vi "UPS_Monitor.vi"() -> ()   [LabVIEW 2021]
doc: "This is the Main VI that performs the UPS and capture data from DAQ and simulate the UPS"
uses:
  Controls/Queue_Operation_Select.ctl
  Controls/Acquired_Data.ctl
  Controls/State_and_Data.ctl
  Controls/Acquired_Datactl_Display.ctl
  Controls/File_Operation_Select.ctl
  Controls/UPS_Data.ctl
  Controls/Notifier_Operation_Select.ctl
  Controls/Error_Data.ctl
panel:
  out "Error_Out":errorcluster
  in  "Error_In":errorcluster
  in  "Tab Control":enum32{"PARAMETER", "DETAILS"}(tab)
  out "ACQUIRED_DATA":T1 {"Power_Consumption" scale=0.0..10.0; "Battery_Power" scale=0.0..100.0}
  out "Low_Power_Indicator":bool caption="Low Power Indicator"
  out "Waveform Graph":dbl[][](graph)
  in  "Record":bool
  in  "Stop":bool
  in  "Pause":bool
  in  "Start":bool
  # "UPS Monitor"
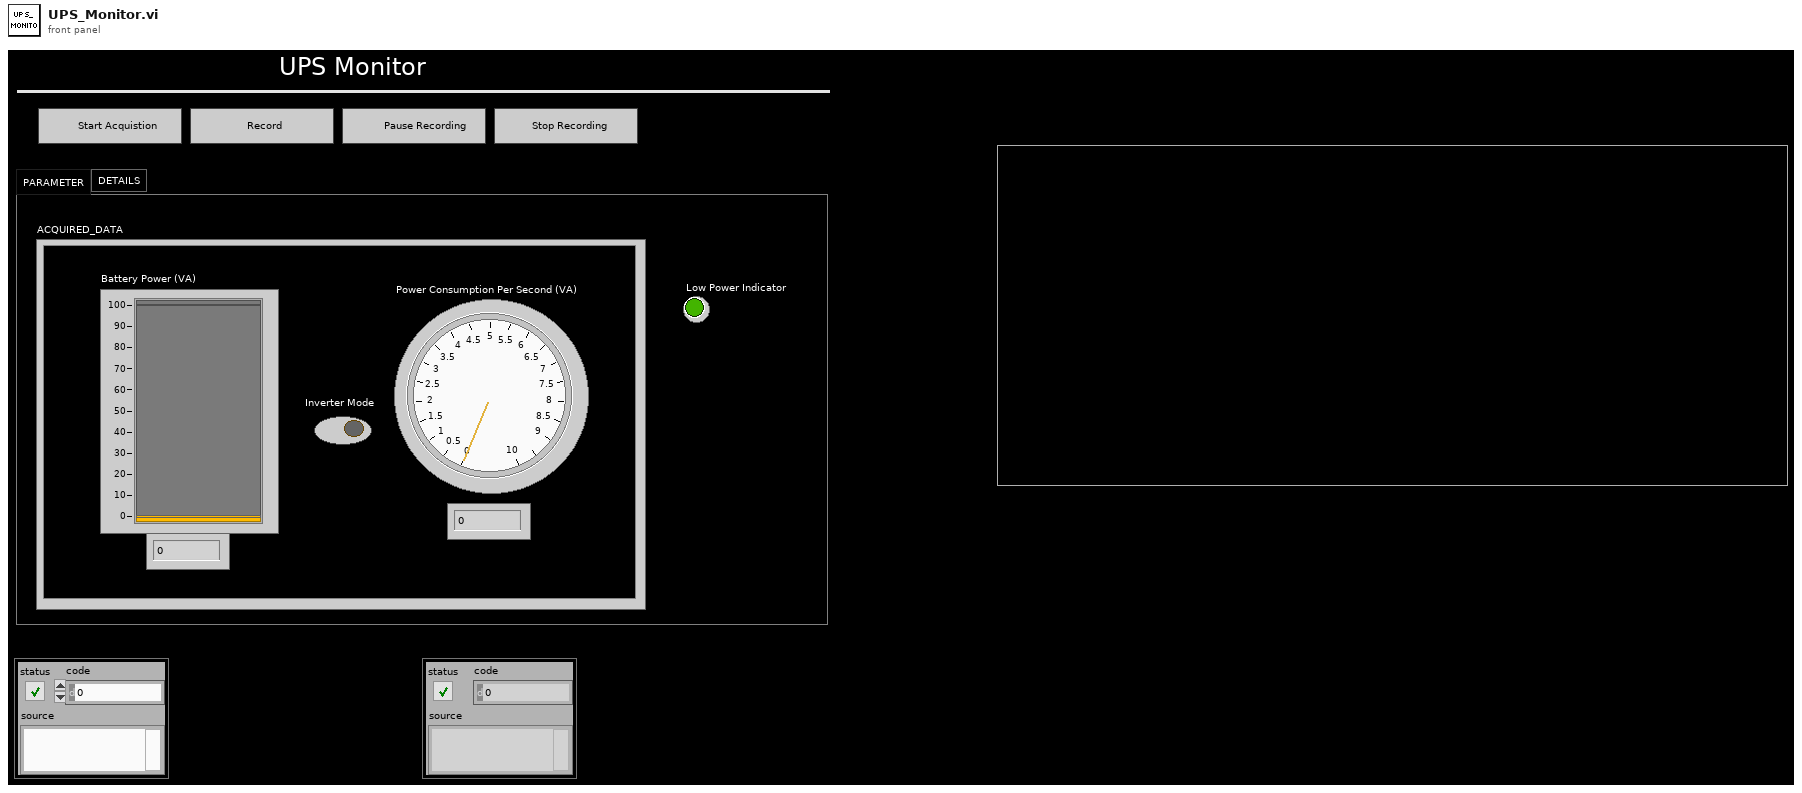
[diagram p1: front panel]
types:
  T1 = typedef "Acquired_Datactl_Display.ctl" = cluster{"Battery_Power":dbl, "Power_Consumption":dbl, "Inverter_Mode":bool}
  T2 = typedef "File_Operation_Select.ctl" = enum16{"Open", "Write", "Read", "Close"}
  T3 = typedef "Queue_Operation_Select.ctl" = enum16{"Obtain_Queue", "Enqueue", "Enqueue_First", "Enqueue_N", "Lossy_Enqueue", "Preview", "Queue_Status", "Dequeue", "Flush", "Release_Queue"}
  T4 = typedef "Notifier_Operation_Select.ctl" = enum16{"Obtain_Notifier", "Send_Notification", "Get_Notifier_Status", "Release_Notifier"}
  T5 = typedef "State_and_Data.ctl" = cluster{"State":string, "Data":variant}
  T6 = typedef "UPS_Data.ctl" = cluster{"ACQUIRED_DATA":T7, "Start":bool, "Pause":bool, "Record":bool, "Low_Power":bool, "Power_and_Power_Consumed":dbl[][], "State_and_Data_In":T5, "File_Path":path, "Application_Directory":path, "Record_Select":enum8{"Enabled", "Disabled", "Disabled and Grayed Out"}, "Stop_Select":enum8{"Enabled", "Disabled", "Disabled and Grayed Out"}}
  T7 = typedef "Acquired_Data.ctl" = cluster{"Battery_Power":dbl, "Power_Consumption":dbl, "Inverter_Mode":bool}
  T8 = enum8{"Enabled", "Disabled", "Disabled and Grayed Out"}
  T9 = typedef "Error_Data.ctl" = cluster{"Module_Name":string, "Error":errorcluster}
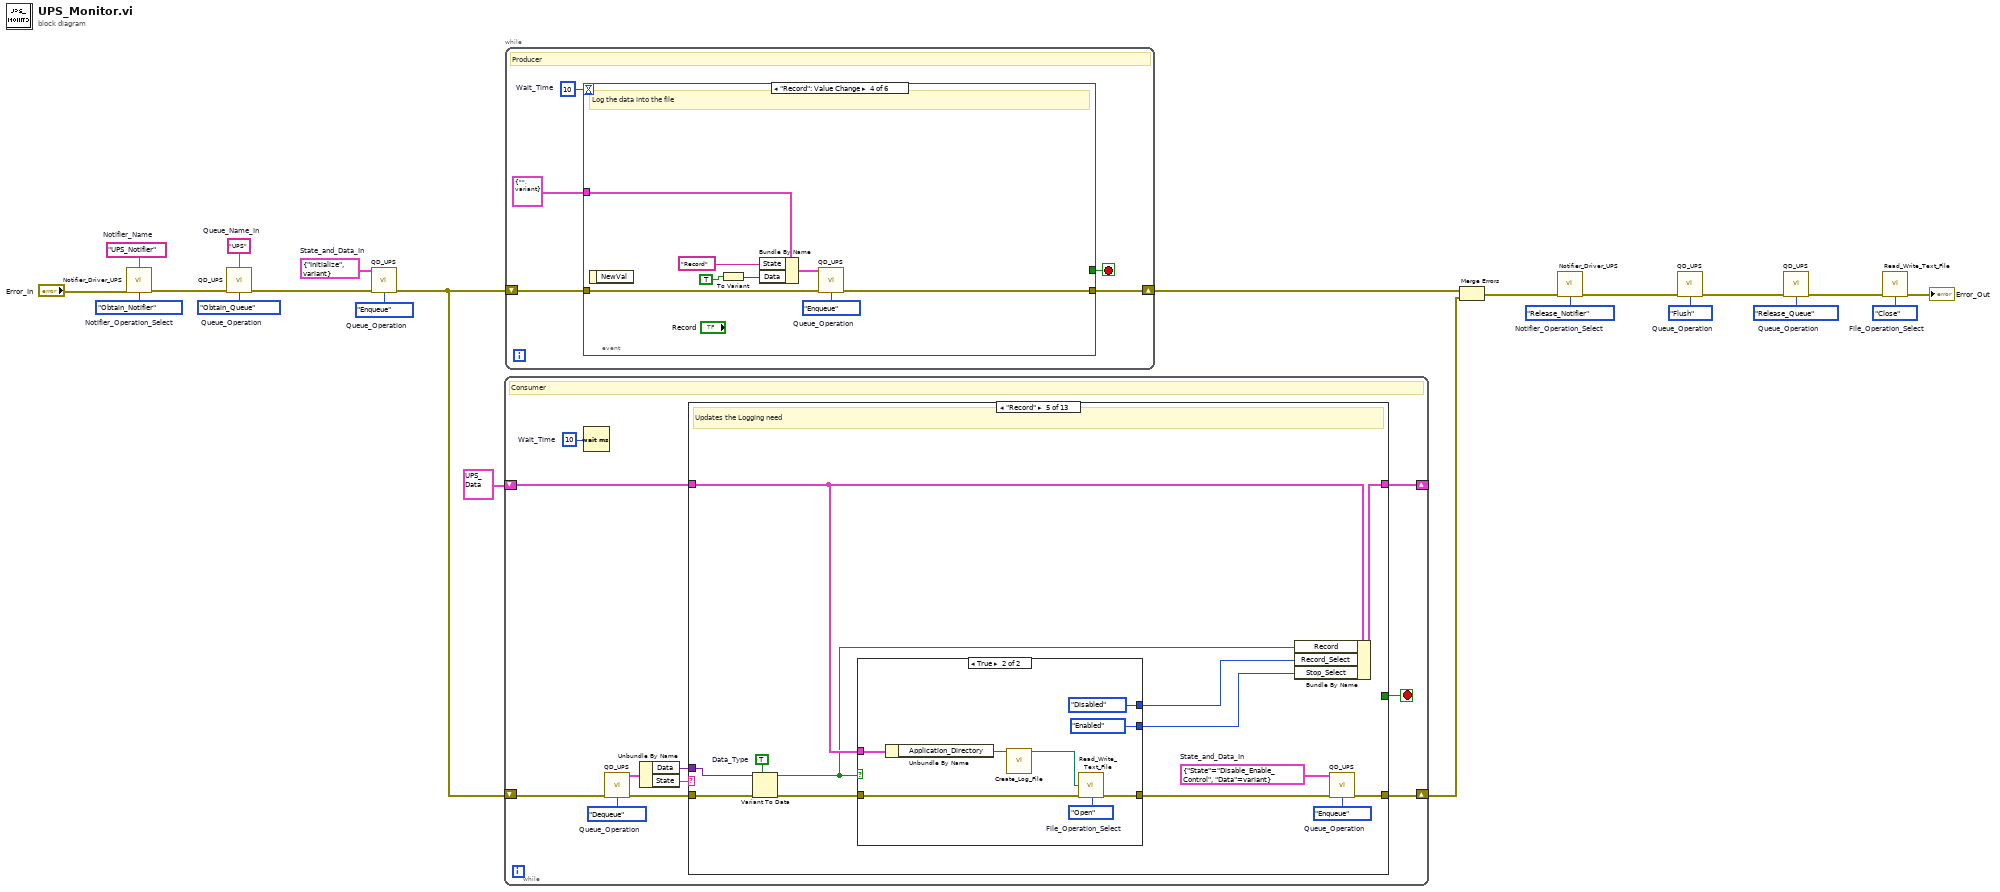
[diagram p0: block diagram]
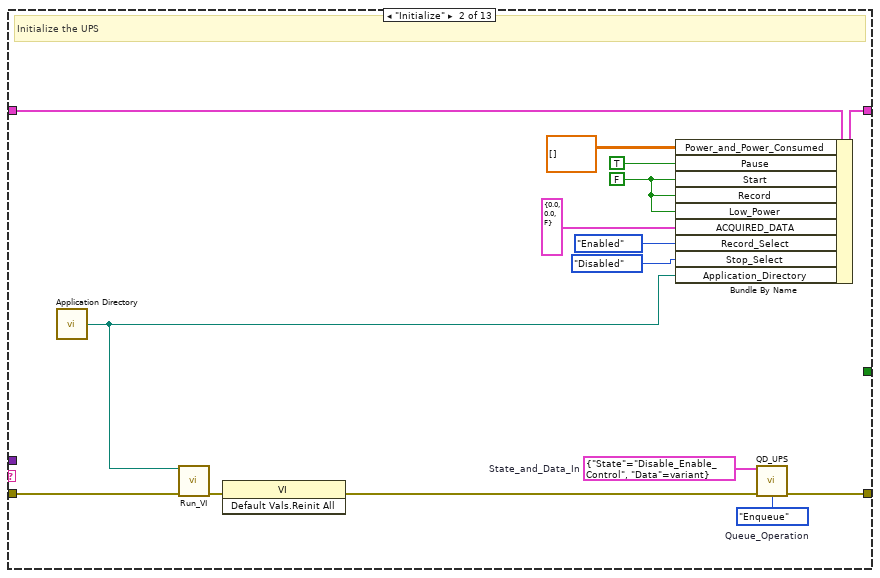
[diagram p3: hidden frame]
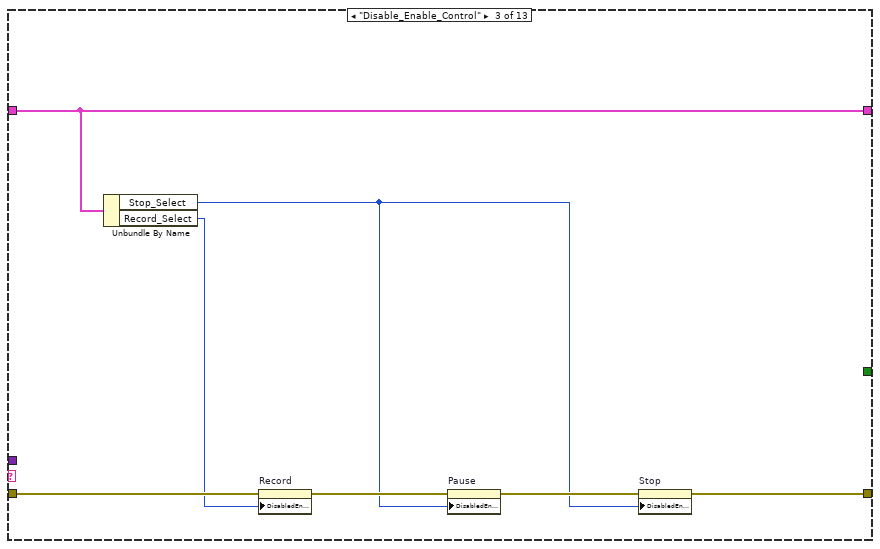
[diagram p4: hidden frame]
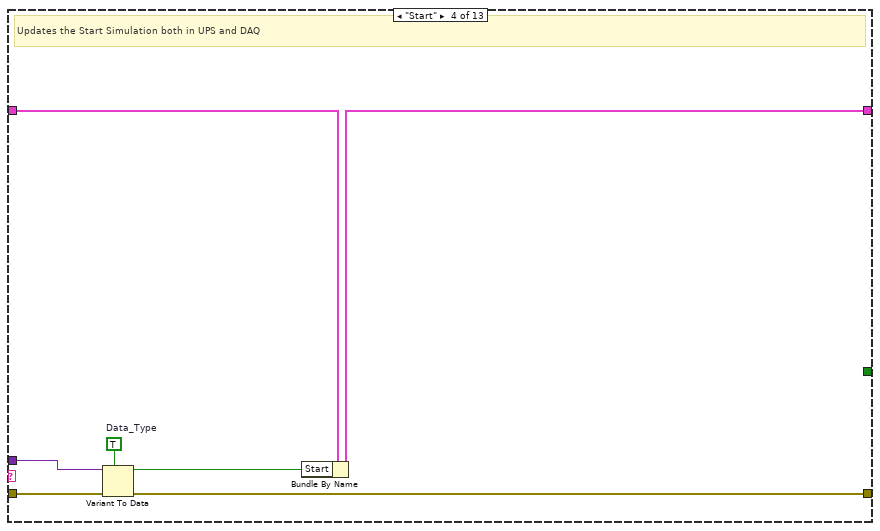
[diagram p5: hidden frame]
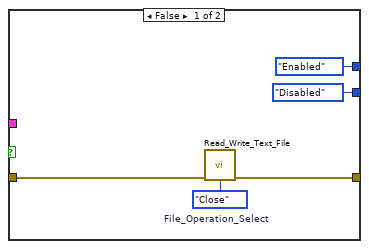
[diagram p6: hidden frame]
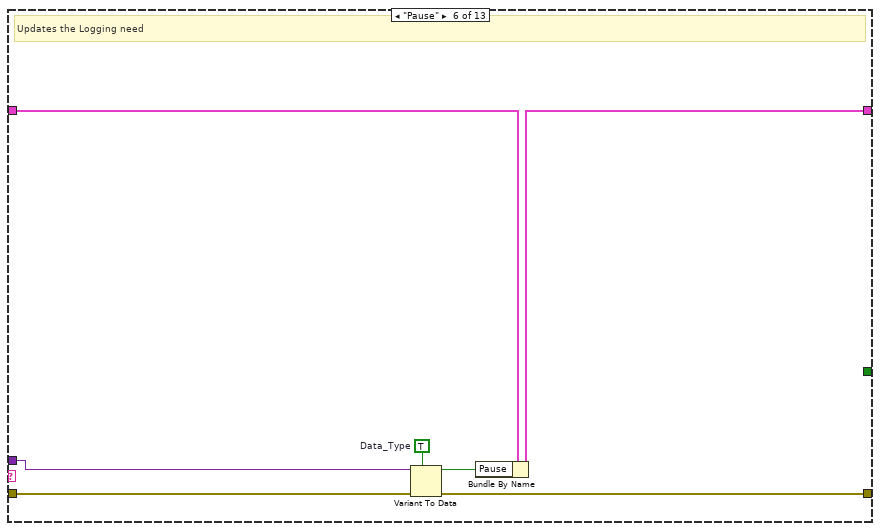
[diagram p7: hidden frame]
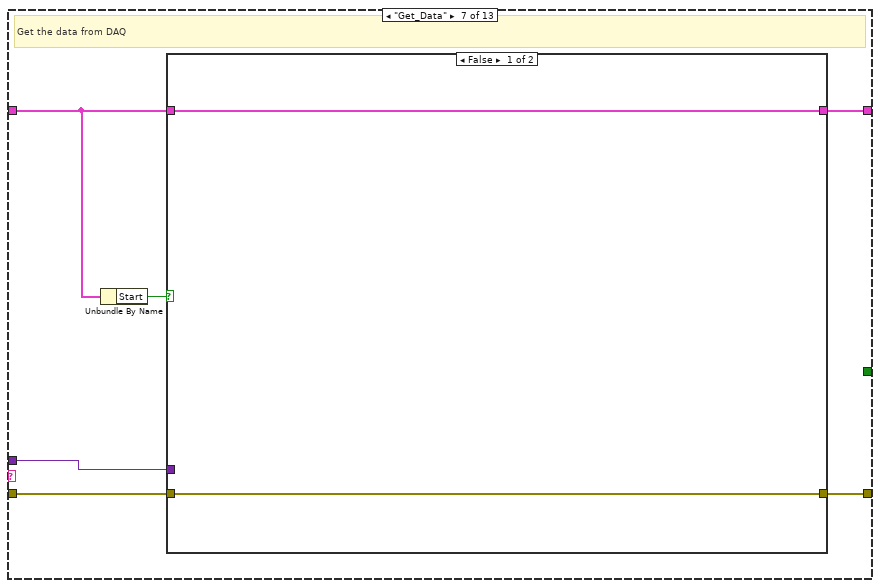
[diagram p8: hidden frame]
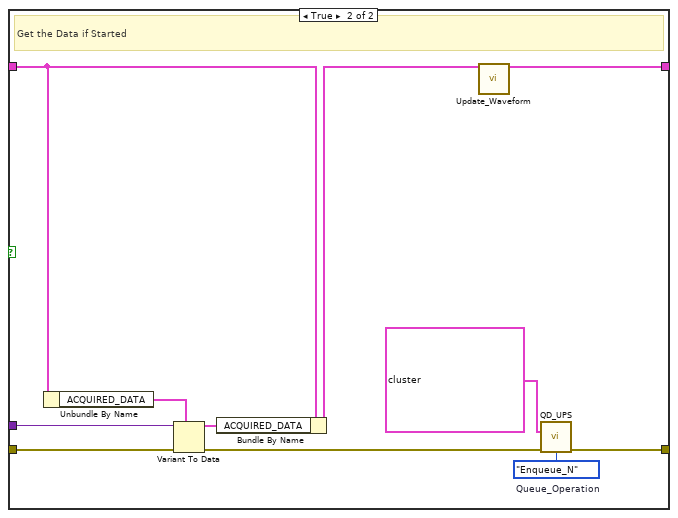
[diagram p9: hidden frame]
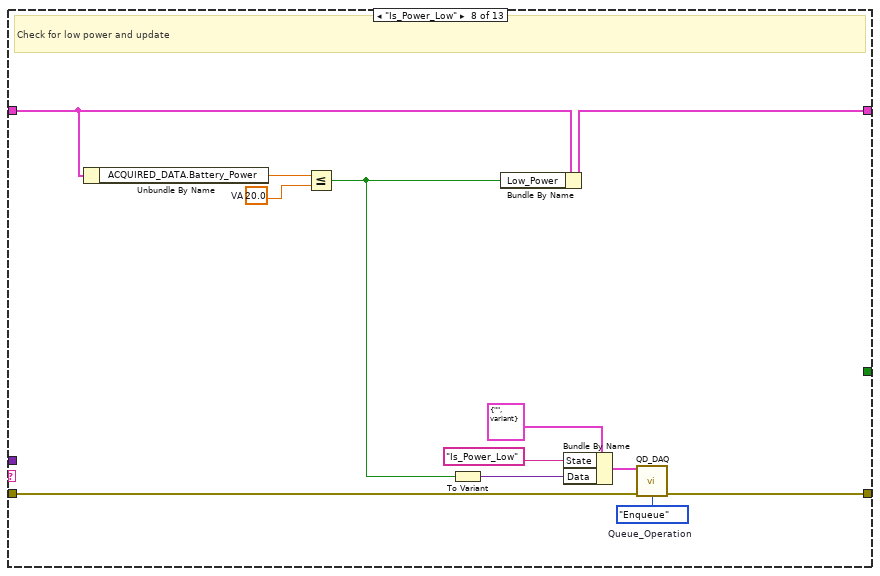
[diagram p10: hidden frame]
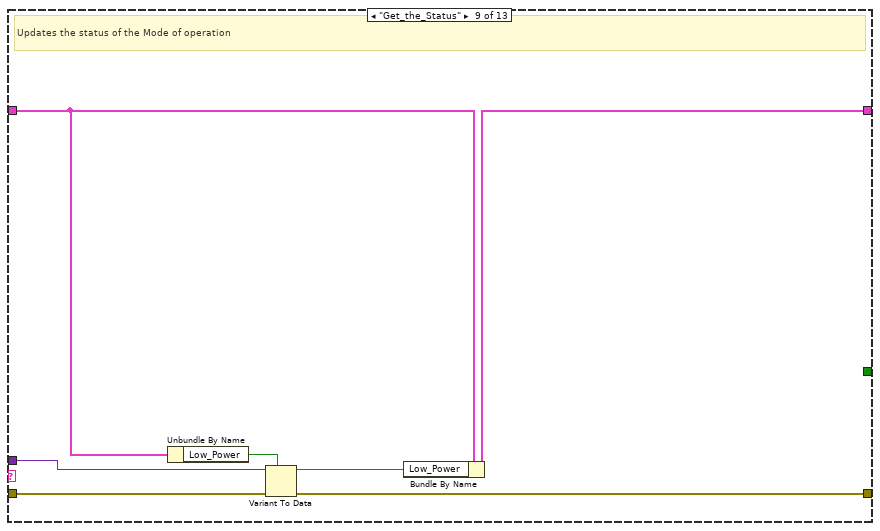
[diagram p11: hidden frame]
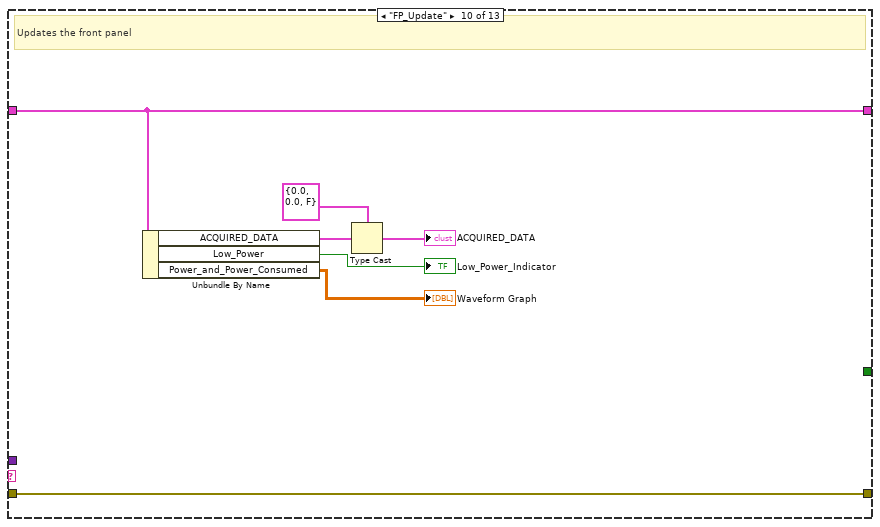
[diagram p12: hidden frame]
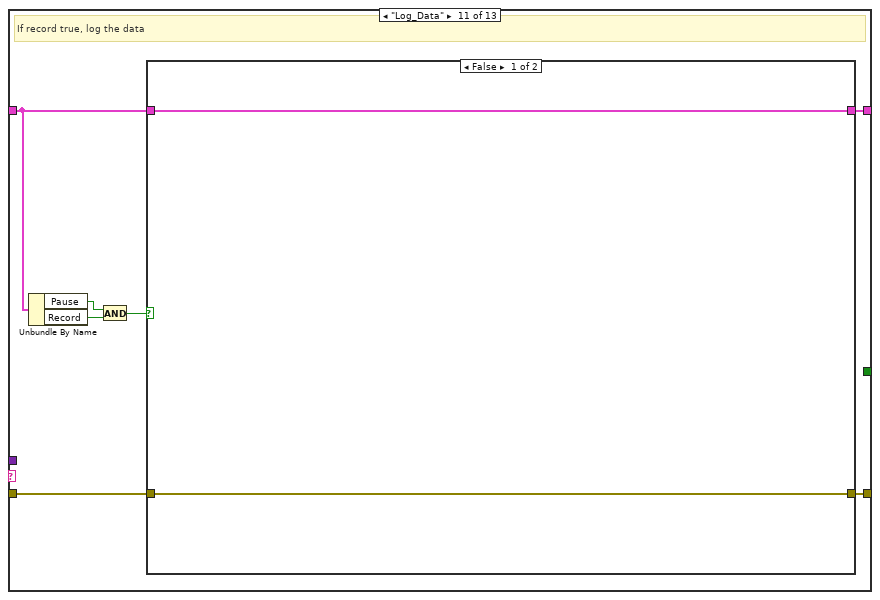
[diagram p13: hidden frame]
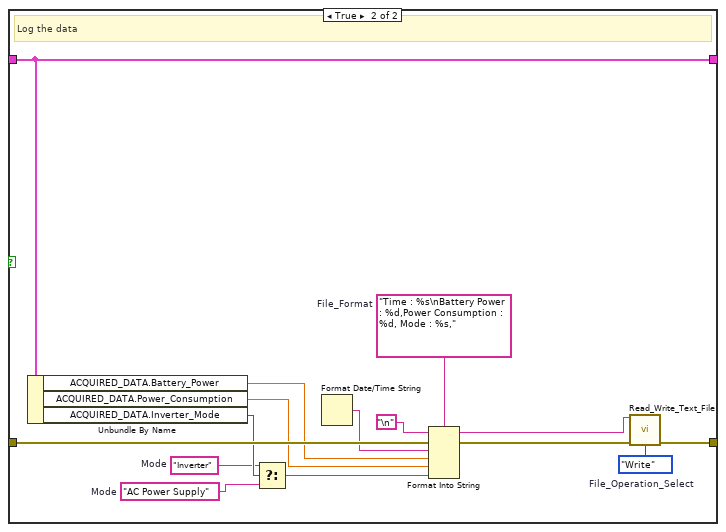
[diagram p14: hidden frame]
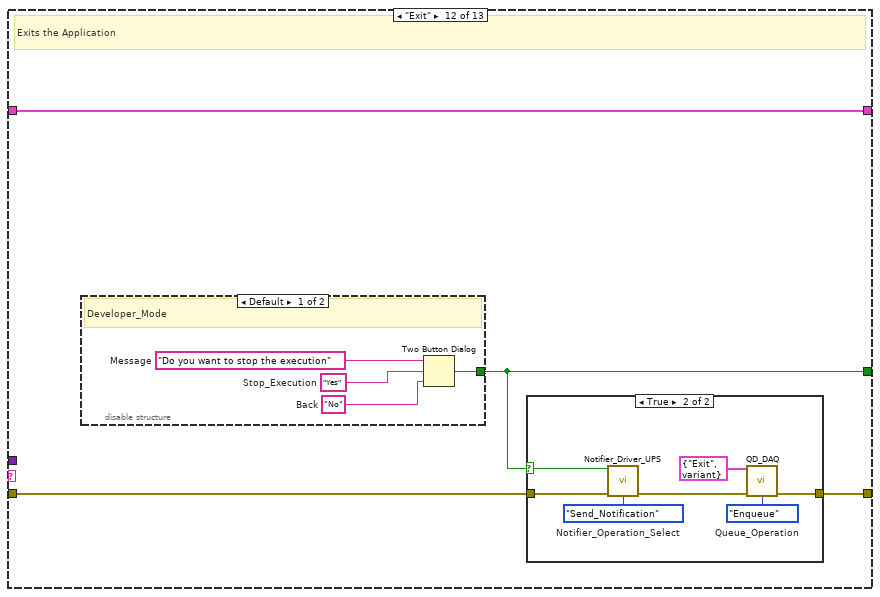
[diagram p15: hidden frame]
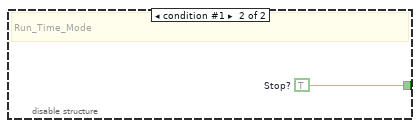
[diagram p17: hidden frame]
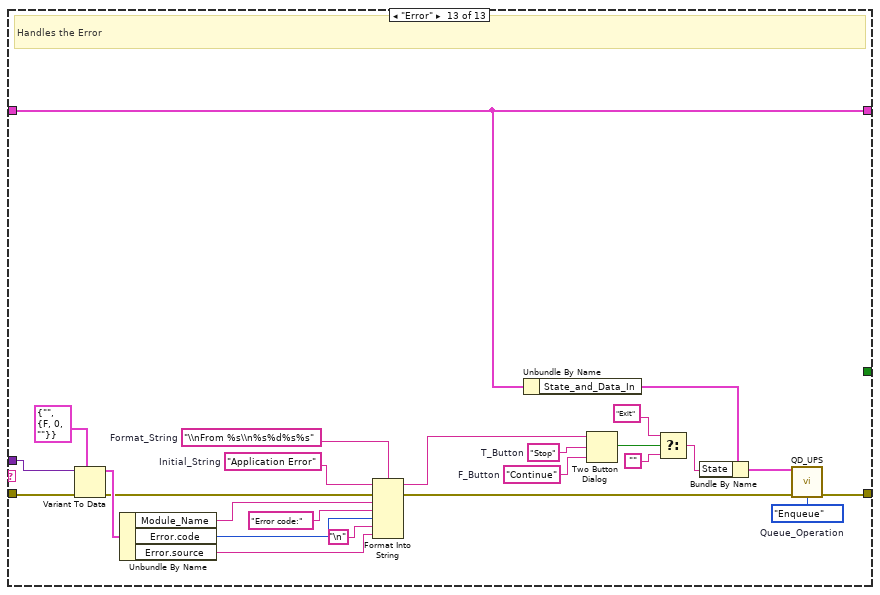
[diagram p18: hidden frame]
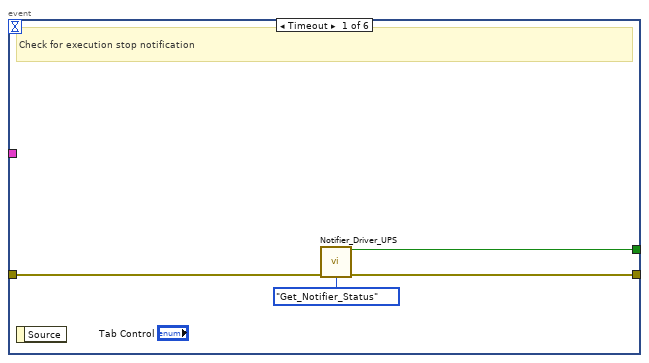
[diagram p19: hidden frame]
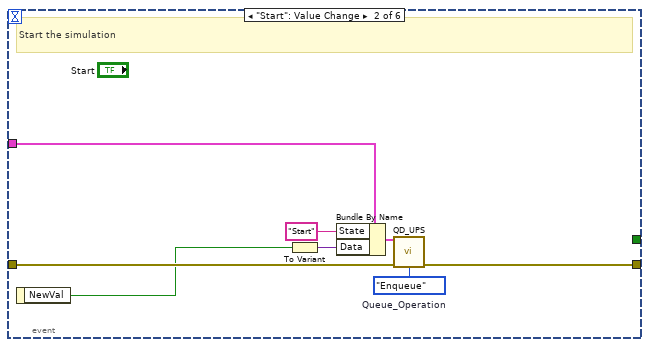
[diagram p20: hidden frame]
diagram:
  w7 = File_Operation_Select."Close"  # File_Operation_Select
  w8 = Queue_Operation_Select."Release_Queue"  # Queue_Operation
  w10 = Queue_Operation_Select."Flush"  # Queue_Operation
  w12 = Notifier_Operation_Select."Release_Notifier"  # Notifier_Operation_Select
  w14 = Notifier_Operation_Select."Obtain_Notifier"  # Notifier_Operation_Select
  w15 = "UPS_Notifier"  # Notifier_Name
  w17 = T5 {"State"="Initialize", "Data"=variant}  # State_and_Data_In
  w18 = Queue_Operation_Select."Enqueue"  # Queue_Operation
  w21 = "UPS"  # Queue_Name_In
  w22 = Queue_Operation_Select."Obtain_Queue"  # Queue_Operation
  n1 = call "Notifier_Driver_UPS.vi"("Notifier_Name"=w15, "Error_In"="Error_In", "Notifier_Operation_Select"=w14) -> ("Error_Out"=w16:errorcluster)  [unwired: 11 in, 1 out]
  n2 = call "QD_UPS.vi"("Queue_Name_In"=w21, "Error_In"=w16, "Queue_Operation"=w22) -> ("Error_Out"=w19:errorcluster)  [unwired: 11 in, 1 out]
  n3 = call "QD_UPS.vi"("State_and_Data_In"=w17, "Error_In"=w19, "Queue_Operation"=w18) -> ("Error_Out"=w2:errorcluster)  [unwired: 11 in, 1 out]
  n4 = while {
    shift-right: [w29] -> _
    shift-left: T6 {"ACQUIRED_DATA"={"Battery_Power"=0.0, "Power_Consumption"=0.0, "Inverter_Mode"=FALSE}, "Start"=TRUE, "Pause"=TRUE, "Record"=TRUE, "Low_Power"=TRUE, "Power_and_Power_Consumed"=[], "State_and_Data_In"={"State"="", "Data"=variant}, "File_Path"=path "", "Application_Directory"=path "", "Record_Select"=enum."Enabled", "Stop_Select"=enum."Enabled"} -> [w28]
    shift-right: [w24] -> w6
    shift-left: w2 -> [w33]
    stop <- w26 stop-if-true
    w23 = u32 10  # Wait_Time
    w25 = Queue_Operation_Select."Dequeue"  # Queue_Operation
    # "Consumer"
    n5 = Wait (ms)(milliseconds to wait=w23) -> ()  [unwired: 1 out]
    n6 = call "QD_UPS.vi"("Error_In"=w33, "Queue_Operation"=w25) -> ("State_and_Data_Out"=w31:T5, "Error_Out"=w32:errorcluster)  [unwired: 12 in]
    n7 = Unbundle By Name(w31) -> ("Data"=w27:variant, "State"=w30:string)
    n8 = case shown="\"Record\"" w30 {
      tunnel: w32 -> [w34 w45 w57 w64 w77 w96 w103 w128 w135 w142 w149 w169 w197]
      tunnel: [w35 w49 w54 w61 w76 w95 w100 w124 w134 w141 w147 w170 w196] -> w29
      tunnel: w28 -> [w35 w50 w54 w59 w73 w97 w99 w127 w130 w141 w146 w170 w196]
      tunnel: [w34 w42 w55 w58 w68 w94 w102 w123 w133 w142 w148 w168 w195] -> w24
      tunnel: w27 -> [_ _ _ w63 w75 w93 w101 _ w132 _ _ _ w192]
      tunnel: [_ _ _ _ _ _ _ _ _ _ _ w167 _] -> w26
      frame Default {
      }
      frame "Initialize" {
        w40 = T5 {"State"="Disable_Enable_Control", "Data"=variant}  # State_and_Data_In
        w41 = Queue_Operation_Select."Enqueue"  # Queue_Operation
        w39 = FALSE ("Start")
        # "Initialize the UPS"
        n9 = call <vilib>:"Application Directory.vi"() -> ("Application Directory"=w37:path)
        n10 = call "Run_VI.vi"("Application_Directory"=w37, "Error_In"=w45) -> ("Error_Out"=w46:errorcluster)  [unwired: 13 in]
        n11 = invoke class="VI" method="Default Vals.Reinit All"(error in=w46) -> (error out=w36:errorcluster)  [unwired: 2 in, 2 out]
        n12 = Bundle By Name(cluster=w50, "Power_and_Power_Consumed"=dbl[][] [], "Pause"=TRUE, "Start"=w39, "Record"=w39, "Low_Power"=w39, "ACQUIRED_DATA"=T7 {"Battery_Power"=0.0, "Power_Consumption"=0.0, "Inverter_Mode"=FALSE}, "Record_Select"=T8."Enabled", "Stop_Select"=T8."Disabled", "Application_Directory"=w37) -> (w49:T6)
        n13 = call "QD_UPS.vi"("State_and_Data_In"=w40, "Error_In"=w36, "Queue_Operation"=w41) -> ("Error_Out"=w42:errorcluster)  [unwired: 11 in, 1 out]
      }
      frame "Disable_Enable_Control" {
        n14 = Unbundle By Name(w54) -> ("Stop_Select"=w51:T8, "Record_Select"=w53:T8)
        n15 = property on="Record" class="Bool (strict)"(error in=w57, "DisabledEnum"=w53) -> (error out=w56:errorcluster)  [unwired: 1 in, 1 out]
        n16 = property on="Pause" class="Bool (strict)"(error in=w56, "DisabledEnum"=w51) -> (error out=w52:errorcluster)  [unwired: 1 in, 1 out]
        n17 = property on="Stop" class="Bool"(error in=w52, "DisabledEnum"=w51) -> (error out=w55:errorcluster)  [unwired: 1 in, 1 out]
      }
      frame "Start" {
        w62 = TRUE  # Data_Type
        # "Updates the Start Simulation both in UPS and DAQ"
        n18 = Variant To Data(error in=w64, type=w62, Variant=w63) -> (data=w60:bool, error out=w58:errorcluster)
        n19 = Bundle By Name(cluster=w59, "Start"=w60) -> (w61:T6)
      }
      frame "Record" {
        w67 = T5 {"State"="Disable_Enable_Control", "Data"=variant}  # State_and_Data_In
        w70 = Queue_Operation_Select."Enqueue"  # Queue_Operation
        w74 = TRUE  # Data_Type
        # "Updates the Logging need"
        n20 = Variant To Data(error in=w77, type=w74, Variant=w75) -> (data=w71:bool, error out=w72:errorcluster)
        n21 = case shown="True" w71 {
          tunnel: w73 -> [_ w90]
          tunnel: [w81 w89] -> w69
          tunnel: w72 -> [w82 w87]
          tunnel: [T8."Disabled" ("Stop_Select") T8."Enabled" ("Stop_Select")] -> w66
          tunnel: [T8."Enabled" ("Record_Select") T8."Disabled" ("Record_Select")] -> w65
          frame False {
            w80 = File_Operation_Select."Close"  # File_Operation_Select
            n22 = call "Read_Write_Text_File.vi"("Error_In"=w82, "File_Operation_Select"=w80) -> ("Error_Out"=w81:errorcluster)  [unwired: 12 in, 1 out]
          }
          frame True {
            w88 = File_Operation_Select."Open"  # File_Operation_Select
            n23 = Unbundle By Name(w90) -> ("Application_Directory"=w86:path)
            n24 = call "Create_Log_File.vi"("Application_Directory"=w86) -> ("New_File_Path"=w83:path)  [unwired: 14 in]
            n25 = call "Read_Write_Text_File.vi"("File_Path"=w83, "Error_In"=w87, "File_Operation_Select"=w88) -> ("Error_Out"=w89:errorcluster)  [unwired: 11 in, 1 out]
          }
        }
        n26 = Bundle By Name(cluster=w73, "Record"=w71, "Record_Select"=w65, "Stop_Select"=w66) -> (w76:T6)
        n27 = call "QD_UPS.vi"("State_and_Data_In"=w67, "Error_In"=w69, "Queue_Operation"=w70) -> ("Error_Out"=w68:errorcluster)  [unwired: 11 in, 1 out]
      }
      frame "Pause" {
        w92 = TRUE  # Data_Type
        # "Updates the Logging need"
        n28 = Variant To Data(error in=w96, type=w92, Variant=w93) -> (data=w91:bool, error out=w94:errorcluster)
        n29 = Bundle By Name(cluster=w97, "Pause"=w91) -> (w95:T6)
      }
      frame "Get_Data" {
        # "Get the data from DAQ"
        n30 = Unbundle By Name(w99) -> ("Start"=w98:bool)
        n31 = case shown="False" w98 {
          tunnel: w103 -> [w104 w116]
          tunnel: [w104 w109] -> w102
          tunnel: w101 -> [_ w114]
          tunnel: w99 -> [w105 w113]
          tunnel: [w105 w106] -> w100
          frame False {
          }
          frame True {
            w108 = Queue_Operation_Select."Enqueue_N"  # Queue_Operation
            # "Get the Data if Started"
            n32 = Unbundle By Name(w113) -> ("ACQUIRED_DATA"=w112:T7)
            n33 = Variant To Data(error in=w116, type=w112, Variant=w114) -> (data=w110:T7, error out=w115:errorcluster)
            n34 = Bundle By Name(cluster=w113, "ACQUIRED_DATA"=w110) -> (w111:T6)
            n35 = call "Update_Waveform.vi"("Data"=w111) -> ("Update_Data"=w106:T6)  [unwired: 14 in]
            n36 = call "QD_UPS.vi"("State_and_Data_N_In"=T5[] [{"State"="Is_Power_Low", "Data"=variant}, {"State"="FP_Update", "Data"=variant}, {"State"="Log_Data", "Data"=variant}], "Error_In"=w115, "Queue_Operation"=w108) -> ("Error_Out"=w109:errorcluster)  [unwired: 11 in, 1 out]
          }
        }
      }
      frame "Is_Power_Low" {
        w121 = Queue_Operation_Select."Enqueue"  # Queue_Operation
        w125 = 20.0  # VA
        # "Check for low power and update"
        n37 = Unbundle By Name(w127) -> ("ACQUIRED_DATA.Battery_Power"=w126:dbl)
        n38 = Less Or Equal?(x=w126, y=w125) -> (x <= y?=w122:bool)
        n39 = To Variant(anything=w122) -> (Variant=w117:variant)
        n40 = Bundle By Name(cluster=w127, "Low_Power"=w122) -> (w124:T6)
        n41 = Bundle By Name(cluster=T5 {"State"="", "Data"=variant} ("Data_In"), "State"="Is_Power_Low", "Data"=w117) -> (w118:T5)
        n42 = call "QD_DAQ.vi"("State_and_Data_In"=w118, "Error_In"=w128, "Queue_Operation"=w121) -> ("Error_Out"=w123:errorcluster)  [unwired: 11 in, 1 out]
      }
      frame "Get_the_Status" {
        # "Updates the status of the Mode of operation"
        n43 = Unbundle By Name(w130) -> ("Low_Power"=w129:bool)
        n44 = Variant To Data(error in=w135, type=w129, Variant=w132) -> (data=w131:bool, error out=w133:errorcluster)
        n45 = Bundle By Name(cluster=w130, "Low_Power"=w131) -> (w134:T6)
      }
      frame "FP_Update" {
        # "Updates the front panel"
        n46 = Unbundle By Name(w141) -> ("ACQUIRED_DATA"=w140:T7, "Low_Power"=→"Low_Power_Indicator":bool, "Power_and_Power_Consumed"=→"Waveform Graph":dbl[][])
        n47 = Type Cast(type=T1 {"Battery_Power"=0.0, "Power_Consumption"=0.0, "Inverter_Mode"=FALSE} ("ACQUIRED_DATA"), x=w140) -> (*(type *) &x=→"ACQUIRED_DATA":T1)
      }
      frame "Log_Data" {
        # "If record true, log the data"
        n48 = Unbundle By Name(w146) -> ("Pause"=w143:bool, "Record"=w145:bool)
        n49 = And(x=w143, y=w145) -> (x .and. y?=w144:bool)
        n50 = case shown="False" w144 {
          tunnel: w146 -> [w151 w160]
          tunnel: w149 -> [w150 w166]
          tunnel: [w150 w165] -> w148
          tunnel: [w151 w160] -> w147
          frame False {
          }
          frame True {
            w155 = "AC Power Supply"  # Mode
            w156 = "Inverter"  # Mode
            w162 = "Time : %s\nBattery Power : %d,Power Consumption : %d, Mode : %s,"  # File_Format
            w164 = File_Operation_Select."Write"  # File_Operation_Select
            # "Log the data"
            n51 = Unbundle By Name(w160) -> ("ACQUIRED_DATA.Battery_Power"=w154:dbl, "ACQUIRED_DATA.Power_Consumption"=w161:dbl, "ACQUIRED_DATA.Inverter_Mode"=w158:bool)
            n52 = Select(t=w156, s=w158, f=w155) -> (s? t:f=w157:string)
            n53 = Format Date/Time String() -> (date/time string=w153:string)  [unwired: 3 in]
            n54 = Format Into String(format string=w162, initial string="\n", error in=w166, w153, w154, w161, w157) -> (resulting string=w152:string, error out=w163:errorcluster)
            n55 = call "Read_Write_Text_File.vi"("Data_In"=w152, "Error_In"=w163, "File_Operation_Select"=w164) -> ("Error_Out"=w165:errorcluster)  [unwired: 11 in, 1 out]
          }
        }
      }
      frame "Exit" {
        # "Exits the Application"
        n56 = disable-structure shown="Default" {
          disable-tunnel: [w179 w183] -> w167
          frame condition #0 (active) {
            w180 = "No"  # Back
            w181 = "Yes"  # Stop_Execution
            w182 = "Do you want to stop the execution"  # Message
            # "Developer_Mode"
            n57 = Two Button Dialog(message=w182, 1:w180, 2:w181) -> (T button?=w179:bool)
          }
          frame condition #1 {
            w183 = TRUE  # Stop?
            # "Run_Time_Mode"
          }
        }
        n58 = case shown="True" w167 {
          selector: w167 -> [_ w172]
          tunnel: w169 -> [w171 w178]
          tunnel: [w171 w177] -> w168
          frame False {
          }
          frame True {
            w173 = Notifier_Operation_Select."Send_Notification"  # Notifier_Operation_Select
            w176 = Queue_Operation_Select."Enqueue"  # Queue_Operation
            n59 = call "Notifier_Driver_UPS.vi"("Notification"=w172, "Error_In"=w178, "Notifier_Operation_Select"=w173) -> ("Error_Out"=w174:errorcluster)  [unwired: 11 in, 1 out]
            n60 = call "QD_DAQ.vi"("State_and_Data_In"=T5 {"State"="Exit", "Data"=variant}, "Error_In"=w174, "Queue_Operation"=w176) -> ("Error_Out"=w177:errorcluster)  [unwired: 11 in, 1 out]
          }
        }
      }
      frame "Error" {
        w193 = Queue_Operation_Select."Enqueue"  # Queue_Operation
        w204 = "\\nFrom %s\\n%s%d%s%s"  # Format_String
        w205 = "Application Error"  # Initial_String
        w206 = "Stop"  # T_Button
        w207 = "Continue"  # F_Button
        # "Handles the Error"
        n61 = Variant To Data(error in=w197, type=T9 {"Module_Name"="", "Error"={"status"=FALSE, "code"=0, "source"=""}} ("Error_Data"), Variant=w192) -> (data=w190:T9, error out=w185:errorcluster)
        n62 = Unbundle By Name(w190) -> ("Module_Name"=w189:string, "Error.code"=w188:i32, "Error.source"=w186:string)
        n63 = Format Into String(format string=w204, initial string=w205, error in=w185, w189, "Error code:" ("input 2"), w188, "\n", w186) -> (resulting string=w208:string, error out=w198:errorcluster)
        n64 = Unbundle By Name(w196) -> ("State_and_Data_In"=w199:T5)
        n65 = Two Button Dialog(message=w208, 1:w207, 2:w206) -> (T button?=w202:bool)
        n66 = Select(t="Exit" ("State"), s=w202, f="") -> (s? t:f=w200:string)
        n67 = Bundle By Name(cluster=w199, "State"=w200) -> (w194:T5)
        n68 = call "QD_UPS.vi"("State_and_Data_In"=w194, "Error_In"=w198, "Queue_Operation"=w193) -> ("Error_Out"=w195:errorcluster)  [unwired: 11 in, 1 out]
      }
    }
  }
  n69 = while {
    shift-right: [w209] -> w5
    shift-left: w2 -> [w213]
    stop <- w212 stop-if-true
    w211 = 10  # Wait_Time
    # "Producer"
    n70 = event shown="[3] \"Record\": Value Change" {
      selector: _ -> [_ _ _ _ _ _]
      dyn-events: _ -> [_ _ _ _ _ _]
      timeout: w211 -> [_ _ _ _ _ _]
      tunnel: w213 -> [w217 w219 w227 w239 w251 w259]
      tunnel: [w216 w220 w228 w235 w244 w258] -> w209
      tunnel: [w214 _ _ _ _ _] -> w212
      tunnel: T5 {"State"="", "Data"=variant} ("State_and_Data_In") -> [_ w225 w234 w237 w249 w256]
      event Timeout {
        # "Check for execution stop notification"
        n71 = event-data() -> ()  [unwired: 1 in, 1 out]
        n72 = call "Notifier_Driver_UPS.vi"("Error_In"=w217, "Notifier_Operation_Select"=Notifier_Operation_Select."Get_Notifier_Status") -> ("Latest_Notification"=w214:bool, "Error_Out"=w216:errorcluster)  [unwired: 12 in]
      }
      event "Start": Value Change {
        w224 = Queue_Operation_Select."Enqueue"  # Queue_Operation
        # "Start the simulation"
        n73 = event-data() -> ("NewVal"=w218:bool)  [unwired: 1 in]
        n74 = To Variant(anything=w218) -> (Variant=w222:variant)
        n75 = Bundle By Name(cluster=w225, "State"="Start", "Data"=w222) -> (w223:T5)
        n76 = call "QD_UPS.vi"("State_and_Data_In"=w223, "Error_In"=w219, "Queue_Operation"=w224) -> ("Error_Out"=w220:errorcluster)  [unwired: 11 in, 1 out]
      }
      event "Pause": Value Change {
        w230 = Queue_Operation_Select."Enqueue"  # Queue_Operation
        # "Pause the simulation"
        n77 = event-data() -> ("NewVal"=w233:bool)  [unwired: 1 in]
        n78 = Not(x=w233) -> (.not. x?=w226:bool)
        n79 = To Variant(anything=w226) -> (Variant=w231:variant)
        n80 = Bundle By Name(cluster=w234, "State"="Pause", "Data"=w231) -> (w232:T5)
        n81 = call "QD_UPS.vi"("State_and_Data_In"=w232, "Error_In"=w227, "Queue_Operation"=w230) -> ("Error_Out"=w228:errorcluster)  [unwired: 11 in, 1 out]
      }
      event "Record": Value Change {
        w242 = Queue_Operation_Select."Enqueue"  # Queue_Operation
        # "Log the data into the file"
        n82 = event-data() -> ()  [unwired: 1 in, 1 out]
        n83 = To Variant(anything=TRUE ("Record")) -> (Variant=w240:variant)
        n84 = Bundle By Name(cluster=w237, "State"="Record", "Data"=w240) -> (w241:T5)
        n85 = call "QD_UPS.vi"("State_and_Data_In"=w241, "Error_In"=w239, "Queue_Operation"=w242) -> ("Error_Out"=w235:errorcluster)  [unwired: 11 in, 1 out]
      }
      event "Stop": Value Change {
        w254 = Queue_Operation_Select."Enqueue"  # Queue_Operation
        # "Stop the execution"
        n86 = event-data() -> ()  [unwired: 1 in, 1 out]
        n87 = To Variant(anything=FALSE ("Stop")) -> (Variant=w252:variant)
        n88 = Bundle By Name(cluster=w249, "State"="Record", "Data"=w252) -> (w253:T5)
        n89 = call "QD_UPS.vi"("State_and_Data_In"=w253, "Error_In"=w251, "Queue_Operation"=w254) -> ("Error_Out"=w247:errorcluster)  [unwired: 11 in, 1 out]
        n90 = property on="Record" class="Bool (strict)"(error in=w247, "Value"=FALSE ("Record")) -> (error out=w246:errorcluster)  [unwired: 1 in, 1 out]
        n91 = property on="Pause" class="Bool (strict)"(error in=w246, "Value"=FALSE ("Pause")) -> (error out=w244:errorcluster)  [unwired: 1 in, 1 out]
      }
      event Panel Close? {
        w257 = Queue_Operation_Select."Enqueue"  # Queue_Operation
        # "Stop the execution"
        n92 = event-data() -> ()  [unwired: 1 in, 4 out]
        n93 = Bundle By Name(cluster=w256, "State"="Exit") -> (w260:T5)
        n94 = call "QD_UPS.vi"("State_and_Data_In"=w260, "Error_In"=w259, "Queue_Operation"=w257) -> ("Error_Out"=w258:errorcluster)  [unwired: 11 in, 1 out]
        n95 = event-data("Discard?"=TRUE) -> ()  [unwired: 1 in, 1 out]
      }
    }
  }
  n96 = Merge Errors(w5, w6) -> (w4:errorcluster)
  n97 = call "Notifier_Driver_UPS.vi"("Error_In"=w4, "Notifier_Operation_Select"=w12) -> ("Error_Out"=w13:errorcluster)  [unwired: 12 in, 1 out]
  n98 = call "QD_UPS.vi"("Error_In"=w13, "Queue_Operation"=w10) -> ("Error_Out"=w11:errorcluster)  [unwired: 12 in, 1 out]
  n99 = call "QD_UPS.vi"("Error_In"=w11, "Queue_Operation"=w8) -> ("Error_Out"=w9:errorcluster)  [unwired: 12 in, 1 out]
  n100 = call "Read_Write_Text_File.vi"("Error_In"=w9, "File_Operation_Select"=w7) -> ("Error_Out"=→"Error_Out":errorcluster)  [unwired: 12 in, 1 out]
